vi "SVT THD and Harmonic Components.vi"   [LabVIEW 2017, in "SoundVib_Distortion.lvlib"]
doc: "Performs a total harmonic distortion analysis, including measuring the fundamental tone and harmonics, and returns the detected fundamental frequency, detected fundamental amplitude, harmonic components, and total harmonic distortion (THD). Wire data to the <B>scaled signal [EU]</B> input to determine the polymorphic instance to use or manually select the instance.\n\nThe following formula calculates THD:\n\nTHD = H / F\n\nwhere H is the harmonic RMS level and F is the fundamental tone RMS level."
uses:
  <vilib>/addons/Sound and Vibration/svt_Distortion/SoundVib_Distortion.lvlib
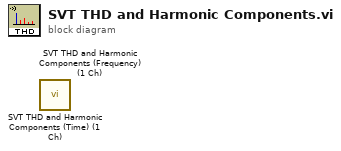
[diagram p0: block diagram]
diagram:
  n1 = call <vilib>:"SVT THD and Harmonic Components (Time) (1 Ch).vi"() -> ()  [unwired: 12 in, 8 out]
  n2 = call <vilib>:"SVT THD and Harmonic Components (Frequency) (1 Ch).vi"() -> ()  [unwired: 12 in, 8 out]
